vi "mod_Complex FFT (Mag-Phase).vi"(0 "Input Data Waveform":T1={"t0"=0.0, "dt"=1.0, "Y"=[]} {"Y" format="%.3f"; "dt" format="%^.2e"; "t0" format="%.4f"}, 7 "dB (on/off)":bool=TRUE, 9 "FFT size":i32=1024) -> (4 "Magnitude":cluster{"f0":dbl, "df":dbl, "Y":dbl[]} {"Y" format="%.2f"; "df" format="%.2f"; "f0" format="%.2f"}, 6 "Phase":dbl[](array[numeric]) format="%.2f")   [LabVIEW 2020, in "niAMT.lvlib"]
uses:
  <vilib>/addons/Modulation/niAMT.lvlib
  <vilib>/addons/Modulation/Analog/controls/Complex Data Waveform.ctl
  <vilib>/Analysis/2dsp.llb/Complex FFT.vi
  <vilib>/measure/NI_MAPro.lvlib
  <vilib>/Analysis/NI_AALPro.lvlib
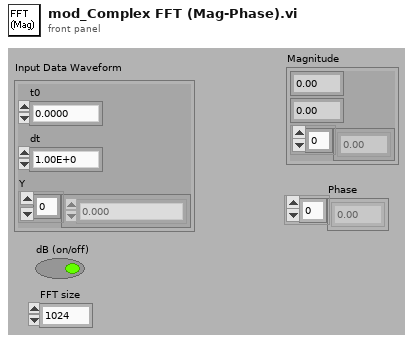
[diagram p1: front panel]
types:
  T1 = typedef "niAMT.lvlib/Complex Data Waveform.ctl" = cluster{"t0":dbl, "dt":dbl, "Y":cdb[]}
  T2 = enum16{"FFT spectrum", "Power spectrum", "Cross spectrum", "Frequency response"}
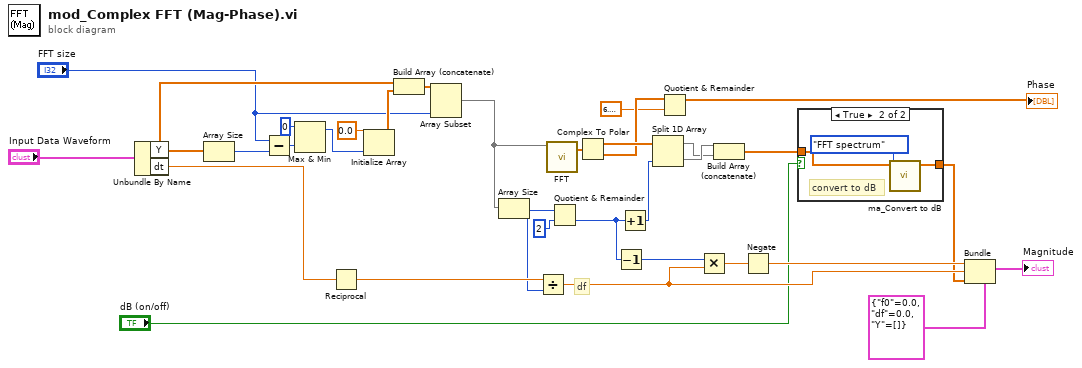
[diagram p0: block diagram]
diagram:
  # "df"
  n1 = Unbundle By Name("Input Data Waveform") -> ("Y"=w9:cdb[], "dt"=w22:dbl)
  n2 = Array Size(array=w9) -> (size(s)=w8:i32)
  n3 = Subtract(x="FFT size", y=w8) -> (x-y=w13:i32)
  n4 = Max & Min(x=0, y=w13) -> (max(x,y)=w11:i32)  [unwired: 1 out]
  n5 = Reciprocal(x=w22) -> (1/x=w32:dbl)
  n6 = Initialize Array(0.0, w11) -> (w14:dbl[])
  n7 = Build Array (concatenate)(w9, w14) -> (w10:cdb[])
  n8 = Array Subset(array=w10, length="FFT size") -> (w1:cdb[])  [unwired: 1 in]
  n9 = Array Size(array=w1) -> (size(s)=w7:i32)
  n10 = Divide(x=w32, y=w7) -> (x/y=w24:dbl)
  n11 = call-poly <vilib>:"FFT.vi"("X"=w1) -> ("FFT {X}"=w33:cdb[])  [unwired: 2 in, 8 out]
  n12 = Quotient & Remainder(x=w7, y=2) -> (floor(x/y)=w5:i32)  [unwired: 1 out]
  n13 = Complex To Polar(r * e^(i*theta)=w33) -> (r=w31:dbl[], theta=w18:dbl[])
  n14 = Decrement(x=w5) -> (x-1=w28:i32)
  n15 = Increment(x=w5) -> (x+1=w27:i32)
  n16 = Split 1D Array(array=w31, index=w27) -> (first subarray=w29:dbl[], second subarray=w30:dbl[])
  n17 = Quotient & Remainder(x=w18, y=6.283185307179586) -> (x-y*floor(x/y)=→"Phase":dbl[])  [unwired: 1 out]
  n18 = Multiply(x=w28, y=w24) -> (x*y=w26:dbl)
  n19 = Build Array (concatenate)(w30, w29) -> (w2:dbl[])
  n20 = Negate(x=w26) -> (-x=w25:dbl)
  n21 = case shown="True" "dB (on/off)" {
    tunnel: w2 -> [w34 w35]
    tunnel: [w34 w37] -> w19
    frame False {
    }
    frame True {
      # "convert to dB"
      n22 = call <vilib>:"ma_Convert to dB.vi"("spectrum type"=T2."FFT spectrum", "spectrum"=w35) -> ("spectrum in dB"=w37:dbl[])  [unwired: 9 out]
    }
  }
  n23 = Bundle(cluster=cluster{"f0":dbl, "df":dbl, "Y":dbl[]} {"f0"=0.0, "df"=0.0, "Y"=[]} ("Magnitude"), "f0"=w25, "df"=w24, "Y"=w19) -> (→"Magnitude":cluster{"f0":dbl, "df":dbl, "Y":dbl[]})
